vi "SENS_IF_FILT_AUTO.vi"(0 "VISA IN":refnum<visa-resource-name>, 1 "AUTO Digital Filter":bool, 5 "error in":errorcluster, 7 "Channel":i32) -> (14 "VISA Out":refnum<visa-resource-name>, 19 "error out":errorcluster)   [LabVIEW 2018, in "PNA-X.lvlib"]
doc: "SENSe<cnum>:IF:FILTer:AUTO <bool> \n(Read-Write) Sets and returns whether the PNA configures the 3-stage digital filter settings or they \nwill be configured manually. When making manual settings, also send SENS:IF:FILT:CMOD OFF \nwhich routes the IF through the 3-stage filter. \nCritical Note \nParameters \n<cnum> Existing channel number. If unspecified, <cnum> is set to 1. \n<bool> (Boolean) \nON (or 1) - Automatic: PNA controls digital filter settings. \nOFF (or 0) - Manual: You control digital filter settings using other Sens:IF \ncommands. \nExamples SENS:IF:FILT:AUTO 1 \nsense2:if:filter:auto 0 \nQuery Syntax SENSe<cnum>:IF:FILTer:AUTO? \nReturn Type Boolean \nDefault ON \nSENSe:IF:FILTer:CMODe <bool> \n(Read-Write) Sets and returns the ADC capture mode modeled as a 2-pole switch in the above \ndiagram. The switch either bypasses or routes the IF through the 3-stage digital filter. \nCritical Note \nParameters \n<bool> (Boolean) \nON (or 1) - The digital filters are bypassed and the raw ADC readings are taken \ndirectly. A maximum of 4096 data points per sweep can be acquired. \nOFF (or 0) - The digital filters are used to process IF information. The filters \ncan be configured automatically or manually using SENS:IF:FILT:AUTO. \nExamples SENS:IF:FILT:CMOD 1 \nsense2:if:filter:cmode 0 \nQuery Syntax SENSe<cnum>:IF:FILTer:CMODe? \n1754\n\nReturn Type Boolean \nDefault OFF"
uses:
  PNA-X.lvlib
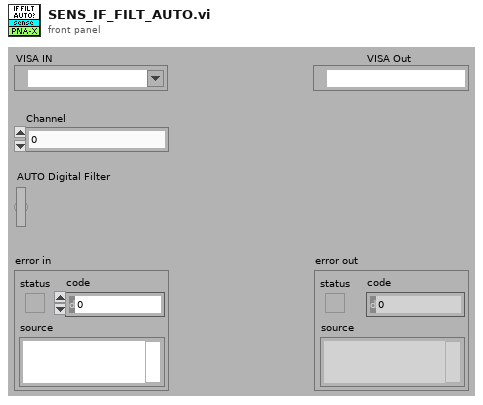
[diagram p1: front panel]
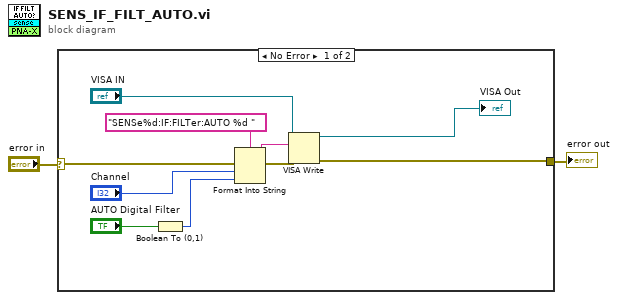
[diagram p0: block diagram]
diagram:
  n1 = case shown="No Error" "error in" {
    selector: "error in" -> [w12 w13]
    tunnel: [w3 w13] -> w1
    frame No Error {
      n2 = Boolean To (0,1)(Boolean="AUTO Digital Filter") -> (0, 1=w5:i16)
      n3 = Format Into String(format string="SENSe%d:IF:FILTer:AUTO %d " ("Cmdline"), error in=w12, "Channel", w5) -> (resulting string=w10:string, error out=w11:errorcluster)  [unwired: 1 in]
      n4 = VISA Write(VISA resource name="VISA IN", write buffer=w10, error in (no error)=w11) -> (VISA resource name out=→"VISA Out":refnum<visa-resource-name>, error out=w3:errorcluster)  [unwired: 1 out]
    }
    frame Error {
    }
  }
  "error out" <- w1
